vi "Scale type.vi"() -> ()   [LabVIEW 2021]
panel:
  in  "Scaling Params 2":dbl[](array[numeric])
  in  "Value 6":dbl
  out "Scaled Value 6":dbl
  in  "Value 5":dbl
  out "Scaled Value 5":dbl
  out "Scaled Value 4":dbl
  in  "Scaling Params":dbl[](array[numeric])
  in  "Value 4":dbl
  out "Scaled Value 3":dbl
  in  "Value 3":dbl
  in  "Value 2":dbl
  out "Scaled Value 2":dbl
  out "Scaled Value":dbl
  in  "Value":dbl
  in  "Coefficients":dbl[](array[numeric])
  out "Used Coefficients":dbl[](array[numeric])
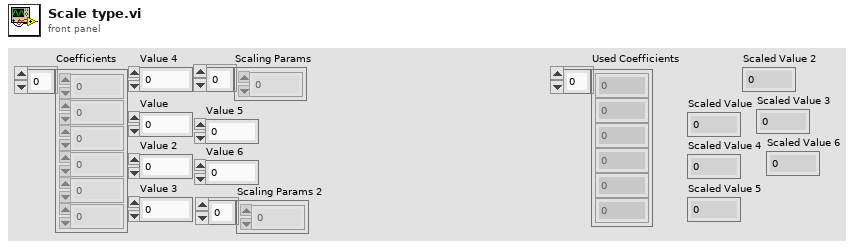
[diagram p1: front panel]
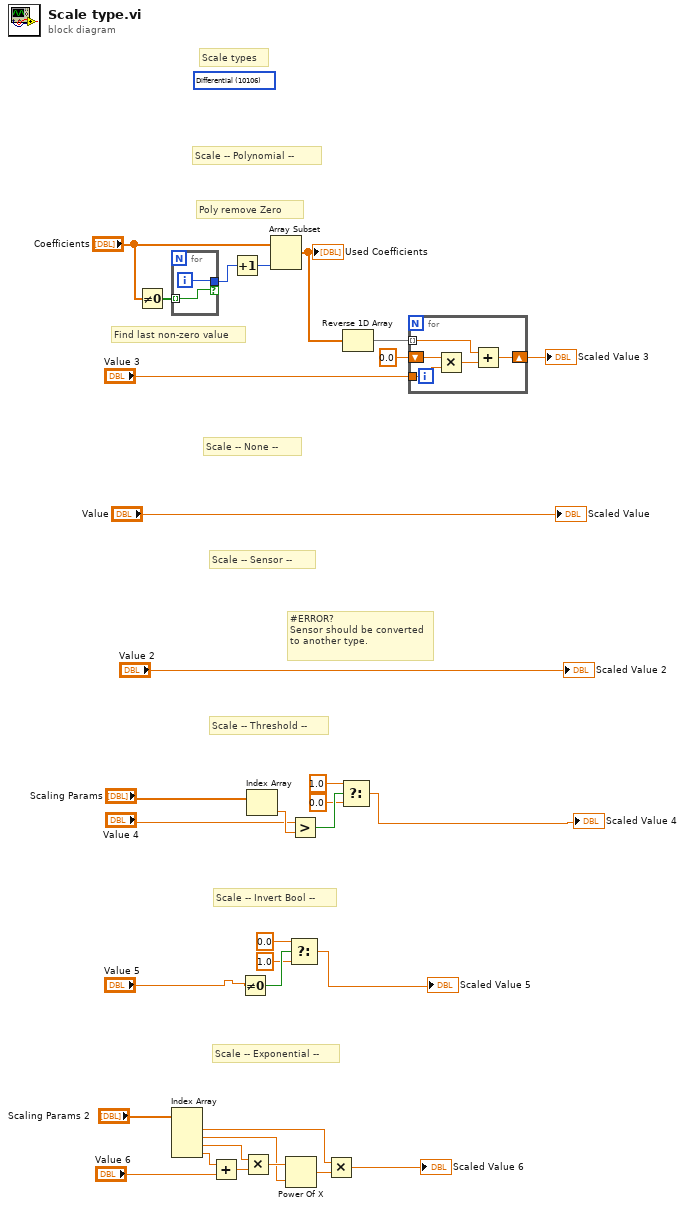
[diagram p0: block diagram]
diagram:
  (unwired) 10106 items=["default"=-1, "RSE"=10083, "NRSE"=10078, "Differential"=10106, "Pseudodifferential"=12529] ("Terminal")
  # "Scale -- Exponential --"
  # "Scale -- Invert Bool --"
  # "Scale -- Threshold --"
  # "#ERROR?\nSensor should be converted to another type."
  # "Scale -- Sensor --"
  # "Scale -- None --"
  # "Scale -- Polynomial --"
  # "Poly remove Zero"
  # "Find last non-zero value"
  # "Scale types"
  n1 = Not Equal To 0?(x="Coefficients") -> (x != 0?=w30:bool[])
  n2 = for {
    tunnel: w30 -> [w34] mode=indexing
    tunnel: [w35] -> w32 if=w34
    i -> [w35]
  }
  n3 = Index Array(array="Scaling Params 2") -> (element #1=w10:dbl, element #2=w4:dbl, element #3=w7:dbl, element #4=w5:dbl)  [unwired: 4 in]
  n4 = Add(x=w5, y="Value 6") -> (x+y=w6:dbl)
  n5 = Increment(x=w32) -> (x+1=w33:i32)
  n6 = Not Equal To 0?(x="Value 5") -> (x != 0?=w15:bool)
  n7 = Multiply(x=w7, y=w6) -> (x*y=w8:dbl)
  n8 = Index Array(array="Scaling Params") -> (element=w19:dbl)  [unwired: 1 in]
  n9 = Array Subset(array="Coefficients", length=w33) -> (w27:dbl[])  [unwired: 1 in]
  "Used Coefficients" <- w27
  n10 = Power Of X(1:w4, 2:w8) -> (0:w9:dbl)
  n11 = Select(t=0.0, s=w15, f=1.0) -> (s? t:f=→"Scaled Value 5":dbl)
  n12 = Greater?(x="Value 4", y=w19) -> (0:w22:bool)
  n13 = Multiply(x=w10, y=w9) -> (x*y=→"Scaled Value 6":dbl)
  n14 = Select(t=1.0, s=w22, f=0.0) -> (s? t:f=→"Scaled Value 4":dbl)
  n15 = Reverse 1D Array(array=w27) -> (reversed array=w28:dbl[])
  n16 = for {
    tunnel: w28 -> [w37] mode=indexing
    tunnel: "Value 3" -> [w39]
    shift-right: [w36] -> w23
    shift-left: 0.0 -> [w40]
    n17 = Multiply(x=w40, y=w39) -> (x*y=w38:dbl)
    n18 = Add(x=w37, y=w38) -> (x+y=w36:dbl)
  }
  "Scaled Value 3" <- w23
  "Scaled Value" <- "Value"
  "Scaled Value 2" <- "Value 2"
